vi "2.2.vi"() -> ()   [LabVIEW 2017]
panel:
  out "2":dbl
  out "3":dbl
  out "1":dbl
  out "Waveform Chart":dbl(graph)
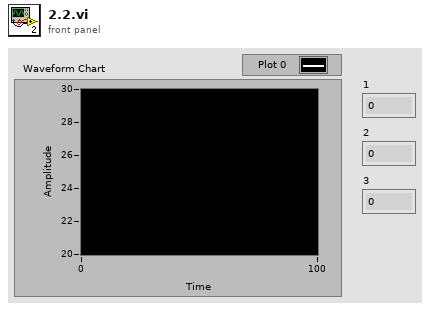
[diagram p1: front panel]
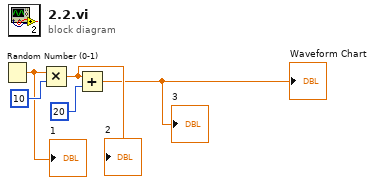
[diagram p0: block diagram]
diagram:
  n1 = Random Number (0-1)() -> (number: 0 to 1=w3:dbl)
  "1" <- w3
  n2 = Multiply(x=w3, y=10) -> (x*y=w2:dbl)
  "2" <- w2
  n3 = Add(x=w2, y=20) -> (x+y=→"Waveform Chart" →"3":dbl)
